vi "TwoLineDistance.vi"(1 "外径下直线":T3, 2 "外径上直线":T3, 3 "Image in":T1) -> (0 "Distance":dbl format="%.2f")   [LabVIEW 2014]
uses:
  <vilib>/vision/Image Controls.llb/IMAQ Image.ctl
  <vilib>/vision/NI_Vision_Development_Module.lvlib
panel:
  out "Perpendicular Line":T2 {"Point 2"."Y" format="%.2f"; "Point 2"."X" format="%.2f"; "Point 1"."Y" format="%.2f"; "Point 1"."X" format="%.2f"}
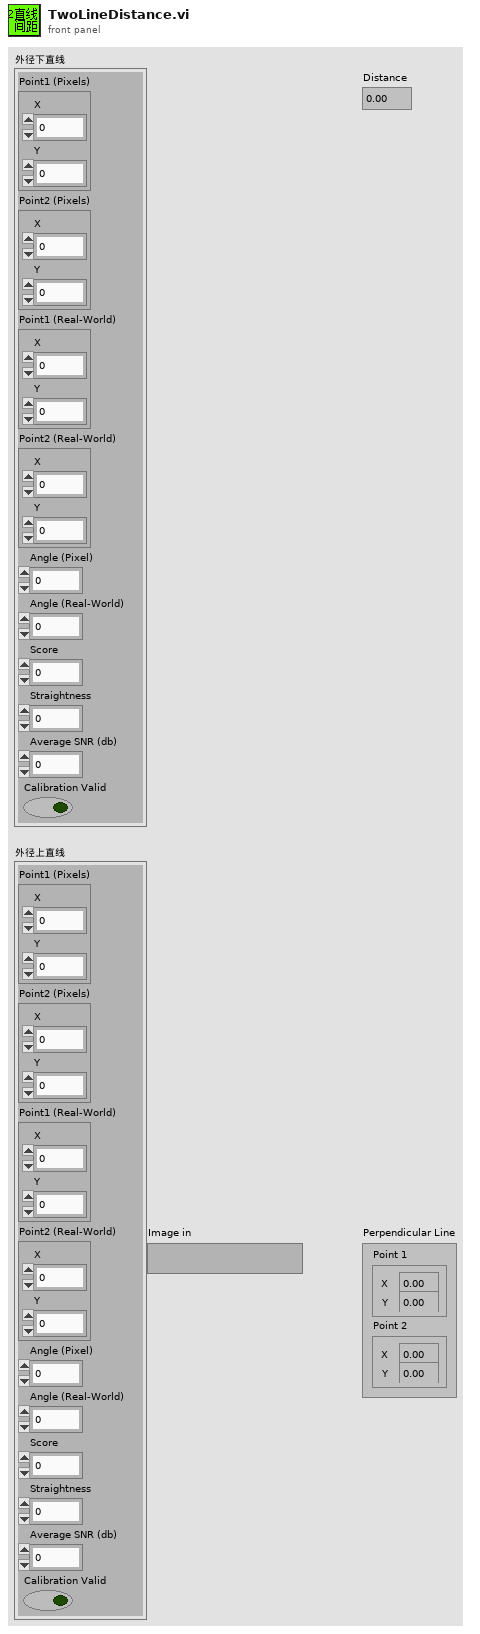
[diagram p1: front panel]
types:
  T1 = typedef "IMAQ Image.ctl" = refnum<image>
  T2 = cluster{"Point 1":cluster{"X":sgl, "Y":sgl}, "Point 2":cluster{"X":sgl, "Y":sgl}}
  T3 = cluster{"Point1 (Pixels)":cluster{"X":sgl, "Y":sgl}, "Point2 (Pixels)":cluster{"X":sgl, "Y":sgl}, "Point1 (Real-World)":cluster{"X":sgl, "Y":sgl}, "Point2 (Real-World)":cluster{"X":sgl, "Y":sgl}, "Angle (Pixel)":dbl, "Angle (Real-World)":dbl, "Score":dbl, "Straightness":dbl, "Average SNR (db)":dbl, "Calibration Valid":bool}
  T4 = cluster{"Point1 (Pixels)":cluster{"X":sgl, "Y":sgl}, "Point2 (Pixels)":cluster{"X":sgl, "Y":sgl}}
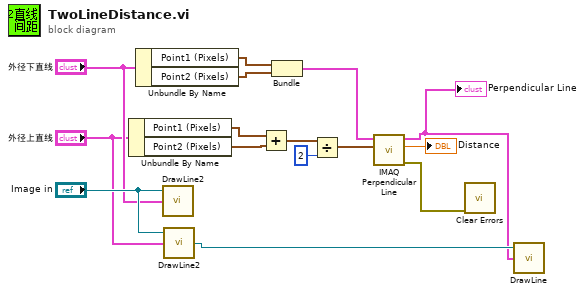
[diagram p0: block diagram]
diagram:
  n1 = Unbundle By Name("外径上直线") -> ("Point1 (Pixels)"=w12:cluster{"X":sgl, "Y":sgl}, "Point2 (Pixels)"=w13:cluster{"X":sgl, "Y":sgl})
  n2 = Unbundle By Name("外径下直线") -> ("Point1 (Pixels)"=w11:cluster{"X":sgl, "Y":sgl}, "Point2 (Pixels)"=w10:cluster{"X":sgl, "Y":sgl})
  n3 = call "DrawLine2.vi"("输入簇"="外径下直线", "img in"="Image in") -> ()  [unwired: 1 in, 1 out]
  n4 = call "DrawLine2.vi"("输入簇"="外径上直线", "img in"="Image in") -> ("Image Out"=w2:T1)  [unwired: 1 in]
  n5 = Add(x=w12, y=w13) -> (x+y=w14:cluster{"X":sgl, "Y":sgl})
  n6 = Bundle("Point1 (Pixels)"=w11, "Point2 (Pixels)"=w10) -> (w8:T4)  [unwired: 1 in]
  n7 = Divide(x=w14, y=2) -> (x/y=w9:cluster{"X":sgl, "Y":sgl})
  n8 = call "IMAQ Perpendicular Line"("Point"=w9, "Line"=w8) -> ("error out"=w6:errorcluster, "Distance"=→"Distance":dbl, "Perpendicular Line"=w1:T2)  [unwired: 7 in]
  "Perpendicular Line" <- w1
  n9 = call <vilib>:"Clear Errors.vi"("error in (no error)"=w6) -> ()  [unwired: 5 in, 2 out]
  n10 = call "DrawLine.vi"("Edge Points"=w1, "img in"=w2) -> ()  [unwired: 1 in, 1 out]
